vi "Configure Measurement Trend Settings.vi"(0 "VISA resource name":refnum<visa-resource-name>, 5 "Trend Vertical":T2, 7 "Trend Smoothing":T1, 11 "error in (no error)":errorcluster) -> (4 "VISA resource name out":refnum<visa-resource-name>, 15 "error out":errorcluster)   [LabVIEW 2009, in "Agilent 8000 Series.lvlib"]
doc: "Configures Measurement Trend analysis and its parameters."
uses:
  Agilent 8000 Series.lvlib
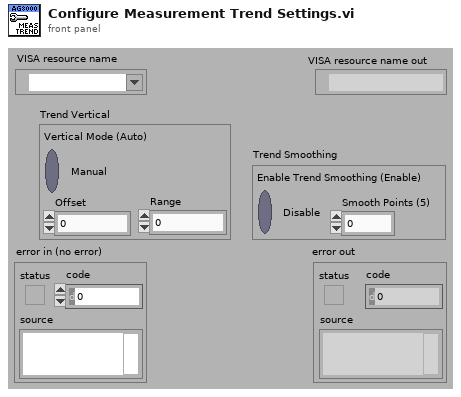
[diagram p1: front panel]
types:
  T1 = cluster{"Enable Trend Smoothing (Enable)":bool, "Smooth Points (5)":dbl}
  T2 = cluster{"Vertical Mode (Auto)":bool, "Offset":dbl, "Range":dbl}
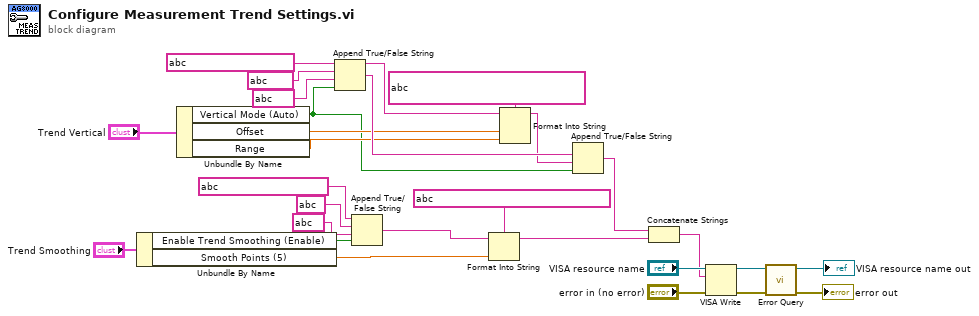
[diagram p0: block diagram]
diagram:
  w7 = string ? ("string (\"\")")
  n1 = Unbundle By Name("Trend Smoothing") -> ("Enable Trend Smoothing (Enable)"=w17:bool, "Smooth Points (5)"=w16:dbl)
  n2 = Unbundle By Name("Trend Vertical") -> ("Vertical Mode (Auto)"=w5:bool, "Offset"=w9:dbl, "Range"=w8:dbl)
  n3 = Append True/False String(1:w5, 2:string ? ("false string"), 3:string ? ("true string"), 4:w7) -> (0:w11:string)
  n4 = Append True/False String(1:w17, 2:string ? ("false string"), 3:string ? ("true string"), 4:string ? ("string (\"\")")) -> (0:w14:string)
  n5 = Format Into String(format string=string ?, initial string=w14, w16) -> (resulting string=w13:string)  [unwired: 1 in, 1 out]
  n6 = Format Into String(format string=string ?, initial string=w7, w9, w8) -> (resulting string=w6:string)  [unwired: 1 in, 1 out]
  n7 = Append True/False String(1:w5, 2:w6, 3:w11) -> (0:w3:string)  [unwired: 1 in]
  n8 = Concatenate Strings(w3, w13) -> (w12:string)
  n9 = VISA Write(VISA resource name="VISA resource name", write buffer=w12, error in (no error)="error in (no error)") -> (VISA resource name out=w26:refnum<visa-resource-name>, error out=w23:errorcluster)  [unwired: 1 out]
  n10 = call "Error Query.vi"("error in (no error)"=w23, "VISA resource name"=w26) -> ("error out"=→"error out":errorcluster, "VISA resource name out"=→"VISA resource name out":refnum<visa-resource-name>)  [unwired: 6 in, 2 out]
